vi "IMG_PARAMS - GetHeight.vi"(8 "error in (no error)":errorcluster, 11 "xiApi.NET.ImgParams":refnum<k24>) -> (0 "error out":errorcluster, 3 "xiApi.NET.ImgParams Out":refnum<k24>, 4 "Height":i32)   [LabVIEW 2013]
doc: "Returns height of the last acquired image."
uses:
  C:/Projects/Cameras3.x/xiLib/xiLIB_64bit/xiLIB/xiCamLib/API/x64/xiApi.NETX64.dll
  xiLIB_64bit/xiLIB/xiCamLib/API/x64/xiApi.NETX64.dll
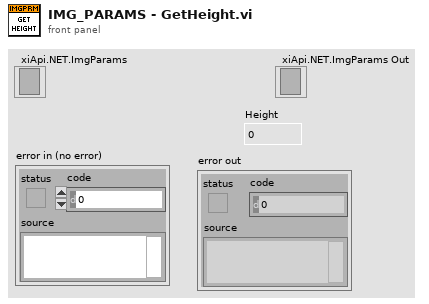
[diagram p1: front panel]
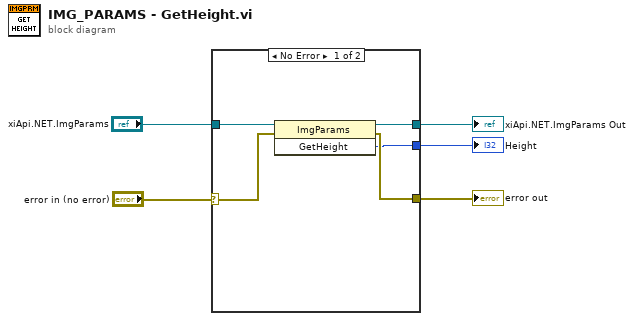
[diagram p0: block diagram]
diagram:
  n1 = case shown="No Error" "error in (no error)" {
    selector: "error in (no error)" -> [w8 w11]
    tunnel: "xiApi.NET.ImgParams" -> [w10 w12]
    tunnel: [w9 w12] -> w4
    tunnel: [w7 w11] -> w2
    tunnel: [w6 _] -> w1
    frame No Error {
      n2 = invoke class="ImgParams" method="GetHeight"(reference=w10, error in=w8) -> (reference out=w9:refnum<k24>, error out=w7:errorcluster, "GetHeight"=w6:i32)  [unwired: 1 in]
    }
    frame Error {
    }
  }
  "xiApi.NET.ImgParams Out" <- w4
  "error out" <- w2
  "Height" <- w1
